vi "Util_Find File in File Path Array.vi"(8 "error in (no error)":errorcluster, 10 "Target file":string, 11 "Files":path[](array[path])) -> (0 "error out":errorcluster, 2 "Found?":bool, 3 "Output Path":path)   [LabVIEW 2016]
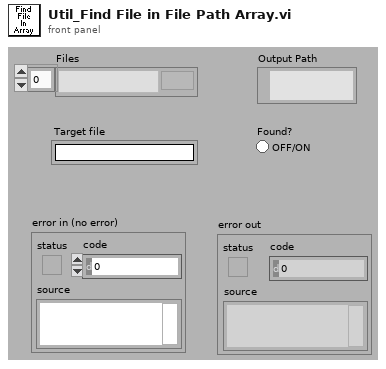
[diagram p1: front panel]
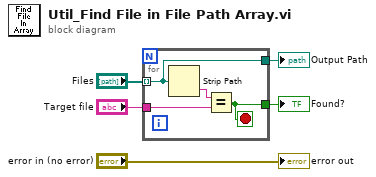
[diagram p0: block diagram]
diagram:
  n1 = for {
    tunnel: "Files" -> [w7] mode=indexing
    tunnel: "Target file" -> [w8]
    tunnel: [w7] -> w5
    tunnel: [w6] -> w2
    stop <- w6 stop-if-true
    n2 = Strip Path(path=w7) -> (name=w9:string)  [unwired: 1 out]
    n3 = Equal?(x=w9, y=w8) -> (x = y?=w6:bool)
  }
  "Output Path" <- w5
  "Found?" <- w2
  "error out" <- "error in (no error)"
